vi "TMDS_clean_and_compress_test.vi"() -> ()   [LabVIEW 2018]
panel:
  out "Seconds for processing":dbl format="%_6g"
  out "Error Out":errorcluster
  in  "error in (no error)":errorcluster
  in  "ZIP file path":path=path "M:/test4/test.zip"
  in  "TDMS File Path":path=path "M:/test4/File1.tdms"
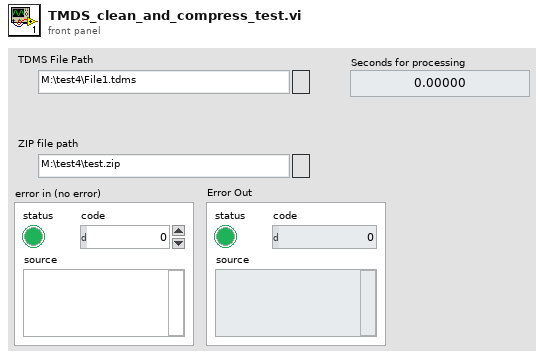
[diagram p1: front panel]
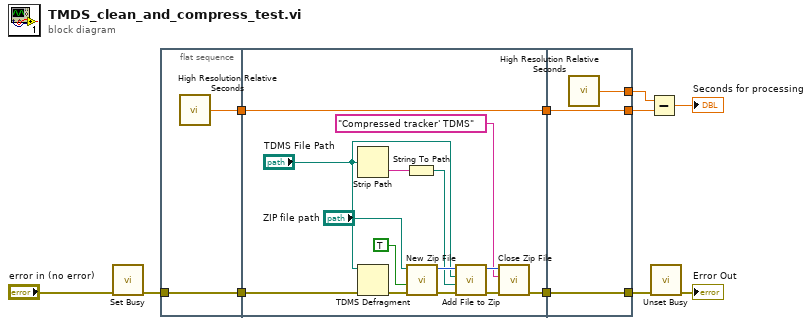
[diagram p0: block diagram]
diagram:
  n1 = call <vilib>:"Set Busy.vi"("error in (no error)"="error in (no error)") -> ("error out"=w4:errorcluster)  [unwired: 9 in, 1 out]
  n2 = flat-sequence {
    tunnel: [w13] -> w10
    tunnel: [w12] -> w5
    tunnel: w4 -> [w12]
    tunnel: [w16] -> w11
    tunnel: w10 -> [w16]
    tunnel: w5 -> [w15]
    tunnel: [w14] -> w2
    tunnel: [w30] -> w8
    tunnel: w11 -> [w30]
    tunnel: [w29] -> w9
    tunnel: [w28] -> w3
    tunnel: w2 -> [w28]
    frame #0 {
      n3 = call <vilib>:"High Resolution Relative Seconds.vi"() -> ("relative seconds"=w13:dbl)
    }
    frame #1 {
      n4 = Strip Path(path="TDMS File Path") -> (name=w19:string)  [unwired: 1 out]
      n5 = TDMS Defragment(4:w15, 7:"TDMS File Path") -> (0:w25:errorcluster)
      n6 = String To Path(string=w19) -> (path=w18:path)
      n7 = call <vilib>:"New Zip File.vi"("error in (no error)"=w25, "confirm overwrite? (F)"=TRUE, "target"="ZIP file path") -> ("error out"=w23:errorcluster, "zip file out"=w24:i64)  [unwired: 2 in, 1 out]
      n8 = call <vilib>:"Add File to Zip.vi"("error in (no error)"=w23, "destination path in zip"=w18, "source file path"="TDMS File Path", "zip file in"=w24) -> ("error out"=w22:errorcluster, "zip file out"=w21:i64)  [unwired: 6 in]
      n9 = call <vilib>:"Close Zip File.vi"("error in (no error)"=w22, "comments"="Compressed tracker' TDMS", "zip file in"=w21) -> ("error out"=w14:errorcluster)  [unwired: 4 in]
    }
    frame #2 {
      n10 = call <vilib>:"High Resolution Relative Seconds.vi"() -> ("relative seconds"=w29:dbl)
    }
  }
  n11 = Subtract(x=w9, y=w8) -> (x-y=→"Seconds for processing":dbl)
  n12 = call <vilib>:"Unset Busy.vi"("error in (no error)"=w3) -> ("error out"=→"Error Out":errorcluster)  [unwired: 10 in]
